vi "WidgetLocation.vi"(6 "error in":errorcluster, 9 "Control in":refnum<class "Control.lvclass">) -> (0 "error out":errorcluster, 3 "Control out":refnum<class "Control.lvclass">, 4 "Bounds":T1, 5 "Location":T2)   [LabVIEW 2014, in "Control.lvclass"]
uses:
  Control.lvclass
  <vilib>/Utility/miscctls.llb/LVPositionTypeDef.ctl
  <vilib>/Utility/miscctls.llb/LVBoundsTypeDef.ctl
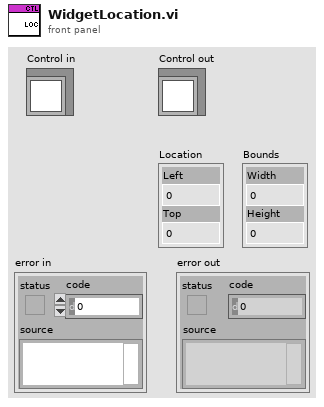
[diagram p1: front panel]
types:
  T1 = typedef "LVBoundsTypeDef.ctl" = cluster{"Width":u32, "Height":u32}
  T2 = typedef "LVPositionTypeDef.ctl" = cluster{"Left":i32, "Top":i32}
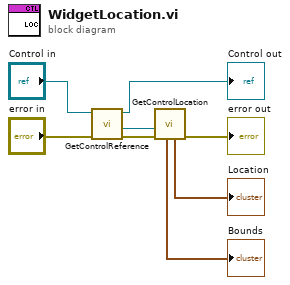
[diagram p0: block diagram]
diagram:
  n1 = call "GetControlReference.vi"("error in"="error in", "Control in"="Control in") -> ("error out"=w5:errorcluster, "control reference"=w4:refnum<vi>, "Control out"=→"Control out":refnum<class "Control.lvclass">)  [unwired: 7 in]
  n2 = call "GetControlLocation.vi"("error in"=w5, "Control in"=w4) -> ("error out"=→"error out":errorcluster, "Position"=→"Location":T2, "Bounds"=→"Bounds":T1)  [unwired: 5 in]
